vi "JKI State selector copy.vi"(9 "Error In (no error)":errorcluster, 11 "State Queue":string) -> (1 "Arguments":string, 2 "Current State":string, 3 "Remaining States":string)   [LabVIEW 2024]
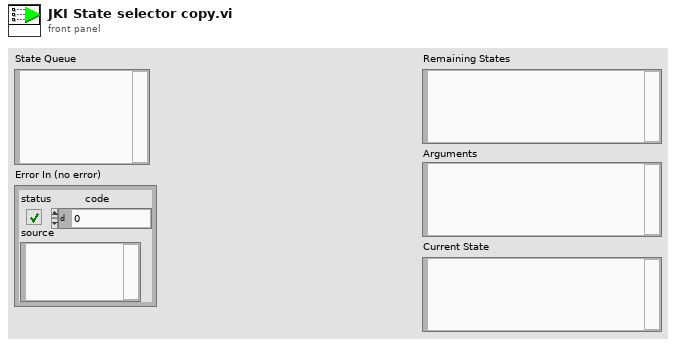
[diagram p1: front panel]
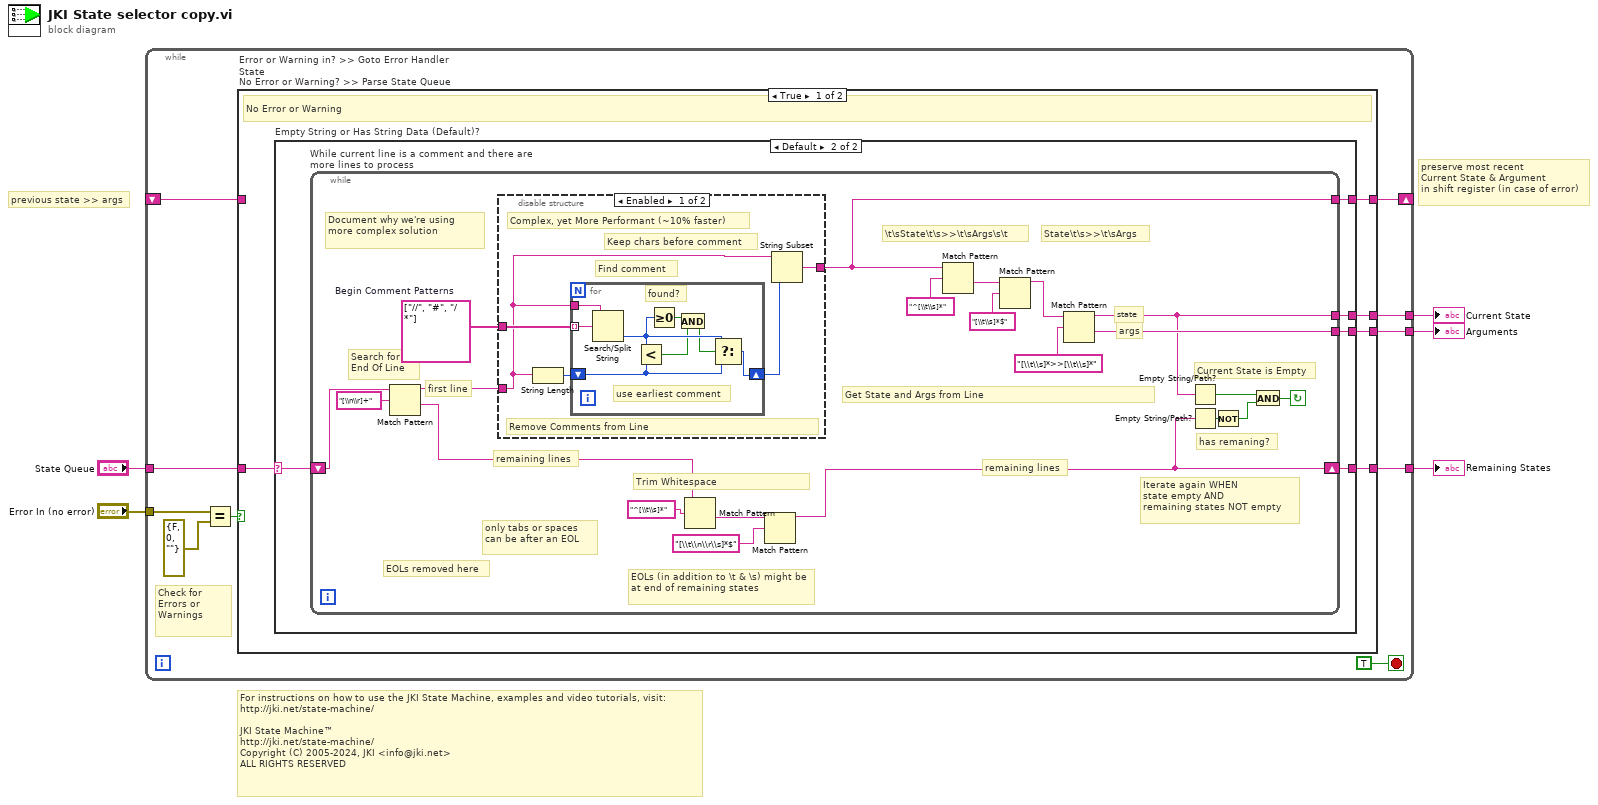
[diagram p0: block diagram]
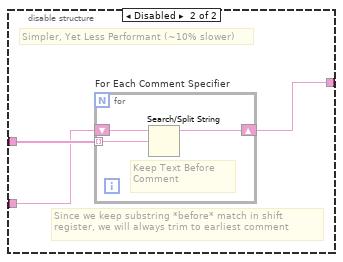
[diagram p3: hidden frame]
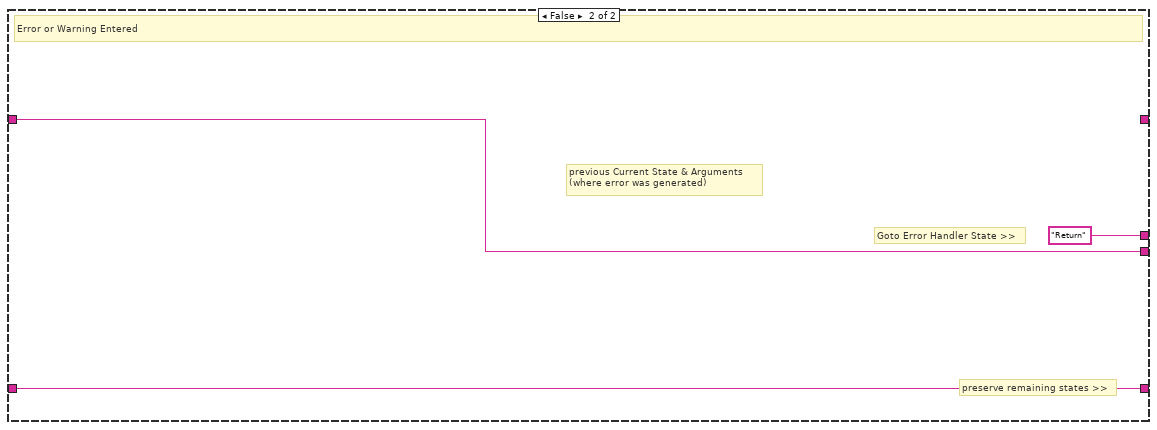
[diagram p4: hidden frame]
diagram:
  # "previous state >> args"
  # "preserve most recent\nCurrent State & Argument\nin shift register (in case of error)"
  # "For instructions on how to use the JKI State Machine, examples and video tutorials, visit:\nhttp://jki.net/state-machine/\n\nJKI State Machine™\nhttp://jki.net/state-machine/\nCopyright (C) 2005-2024, JKI <info@jki.net>\nALL RIGHTS RESERVED"
  n1 = while {
    tunnel: [w15] -> w5
    tunnel: "Error In (no error)" -> [w8]
    tunnel: "State Queue" -> [w13]
    shift-right: [w11] -> _
    shift-left: _ -> [w10]
    tunnel: [w14] -> w3
    tunnel: [w9] -> w1
    stop <- TRUE stop-if-true
    # "Check for Errors or Warnings"
    n2 = Equal?(x=w8, y=errorcluster {"status"=FALSE, "code"=0, "source"=""} ("error constant")) -> (x = y?=w6:bool)
    n3 = case "Error or Warning in? >> Goto Error Handler State\nNo Error or Warning? >> Parse State Queue" shown="True" w6 {
      tunnel: [w18 w68] -> w15
      tunnel: [w20 "Return"] -> w14
      tunnel: [w19 w66] -> w9
      tunnel: w13 -> [w17 w68]
      tunnel: [w16 _] -> w11
      tunnel: w10 -> [_ w66]
      frame True {
        # "No Error or Warning"
        n4 = case "Empty String or Has String Data (Default)?" shown="Default" w17 {
          selector: w17 -> [_ w22]
          tunnel: [_ w25] -> w20
          tunnel: [_ w24] -> w19
          tunnel: [_ w23] -> w18
          tunnel: [_ w21] -> w16
          frame "" {
            # "Do Nothing if Empty String"
            # "<< Wiring into the Case Selector is much more performant than using \"Empty String/Path?\" primitive"
          }
          frame Default {
            n5 = while "While current line is a comment and there are more lines to process" {
              tunnel: [w45] -> w25
              tunnel: [w46] -> w24
              shift-right: [w41] -> w23
              shift-left: w22 -> [w39]
              tunnel: [w26] -> w21
              stop <- w42 continue-if-true
              w38 = string[] ["//", "#", "/*"]  # Begin Comment Patterns
              # "Get State and Args from Line"
              # "State\\t\\s>>\\t\\sArgs"
              # "\\t\\sState\\t\\s>>\\t\\sArgs\\s\\t"
              # "remaining lines"
              # "EOLs (in addition to \\t & \\s) might be at end of remaining states"
              # "Document why we're using more complex solution"
              # "Trim Whitespace"
              # "EOLs removed here"
              # "only tabs or spaces can be after an EOL"
              # "Current State is Empty"
              # "has remaning?"
              # "remaining lines"
              # "first line"
              # "Search for End Of Line"
              # "Iterate again WHEN\nstate empty AND\nremaining states NOT empty"
              # "args"
              # "state"
              n6 = Match Pattern(string=w39, regular expression="[\\n\\r]+") -> (before substring=w37:string, after substring=w29:string)  [unwired: 1 in, 2 out]
              n7 = disable-structure shown="Enabled" {
                disable-tunnel: w38 -> [w51 w62]
                disable-tunnel: [w50 w61] -> w26
                disable-tunnel: w37 -> [w49 w60]
                frame Enabled {
                  # "Remove Comments from Line"
                  # "Complex, yet More Performant (~10% faster)"
                  # "Keep chars before comment"
                  # "Find comment"
                  n8 = String Length(string=w49) -> (length=w48:i32)
                  n9 = for {
                    tunnel: w51 -> [w56] mode=indexing
                    shift-right: [w58] -> w47
                    shift-left: w48 -> [w59]
                    tunnel: w49 -> [w57]
                    # "found?"
                    # "use earliest comment"
                    n10 = Search/Split String(string=w57, search string/char (-)=w56) -> (offset of match=w55:i32)  [unwired: 1 in, 2 out]
                    n11 = Less?(x=w55, y=w59) -> (x < y?=w53:bool)
                    n12 = Greater Or Equal To 0?(x=w55) -> (x >= 0?=w54:bool)
                    n13 = And(x=w54, y=w53) -> (x .and. y?=w52:bool)
                    n14 = Select(t=w55, s=w52, f=w59) -> (s? t:f=w58:i32)
                  }
                  n15 = String Subset(string=w49, length (rest)=w47) -> (substring=w50:string)  [unwired: 1 in]
                }
                frame Disabled {
                  # "Since we keep substring *before* match in shift register, we will always trim to earliest comment"
                  # "Simpler, Yet Less Performant (~10% slower)"
                  n16 = for "For Each Comment Specifier" {
                    tunnel: w62 -> [w64] mode=indexing
                    shift-right: [w63] -> w61
                    shift-left: w60 -> [w65]
                    # "Keep Text Before Comment"
                    n17 = Search/Split String(string=w65, search string/char (-)=w64) -> (substring before match=w63:string)  [unwired: 1 in, 2 out]
                  }
                }
              }
              n18 = Match Pattern(string=w29, regular expression="^[\\t\\s]*") -> (after substring=w28:string)  [unwired: 1 in, 3 out]
              n19 = Match Pattern(string=w28, regular expression="[\\t\\n\\r\\s]*$") -> (before substring=w41:string)  [unwired: 1 in, 3 out]
              n20 = Match Pattern(string=w26, regular expression="^[\\t\\s]*") -> (after substring=w27:string)  [unwired: 1 in, 3 out]
              n21 = Match Pattern(string=w27, regular expression="[\\t\\s]*$") -> (before substring=w31:string)  [unwired: 1 in, 3 out]
              n22 = Match Pattern(string=w31, regular expression="[\\t\\s]*>>[\\t\\s]*") -> (before substring=w45:string, after substring=w46:string)  [unwired: 1 in, 2 out]
              n23 = Empty String/Path?(string/path=w45) -> (empty?=w44:bool)
              n24 = Empty String/Path?(string/path=w41) -> (empty?=w43:bool)
              n25 = Not(x=w43) -> (.not. x?=w36:bool)
              n26 = And(x=w44, y=w36) -> (x .and. y?=w42:bool)
            }
          }
        }
      }
      frame False {
        # "previous Current State & Arguments\n(where error was generated)"
        # "Goto Error Handler State >>"
        # "preserve remaining states >>"
        # "Error or Warning Entered"
      }
    }
  }
  "Remaining States" <- w5
  "Arguments" <- w1
  "Current State" <- w3
